vi "Insert Data Point.vi"(4 "Error In":errorcluster, 6 "Instance Name":T1, 7 "Data":T2) -> (0 "Error Out":errorcluster)   [LabVIEW 2015, in "Temperature Controller Data Buffer.lvlib"]
uses:
  Temperature Controller Data Buffer.lvlib
  _libraries/Startup Processes/_typedefs/Subpanel Names.ctl
  _libraries/Startup Processes/Startup Processes.lvlib
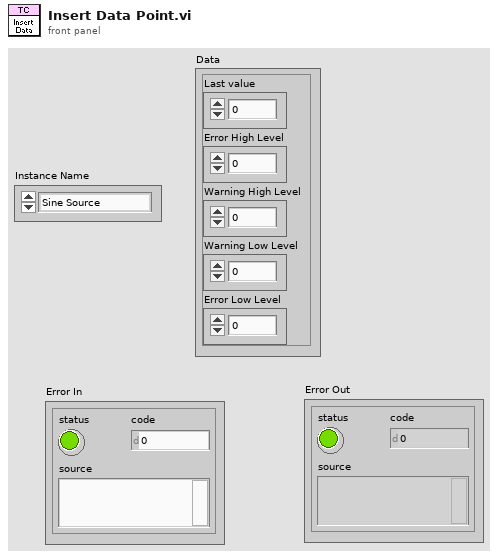
[diagram p1: front panel]
types:
  T1 = typedef "Startup Processes.lvlib/Subpanel Names.ctl" = enum16{"Sine Source", "Ramp Source", "Hen House TC", "Dog House TC", "Out House TC"}
  T2 = cluster{"Last value":dbl, "Error High Level":dbl, "Warning High Level":dbl, "Warning Low Level":dbl, "Error Low Level":dbl}
  T3 = typedef "Temperature Controller Data Buffer.lvlib/buffer data typedef.ctl" = cluster{"TC Data":cluster{"Last value":dbl, "Error High Level":dbl, "Warning High Level":dbl, "Warning Low Level":dbl, "Error Low Level":dbl}[], "Counter":i32}
  T4 = cluster{"Last value":dbl, "Error High Level":dbl, "Warning High Level":dbl, "Warning Low Level":dbl, "Error Low Level":dbl}[]
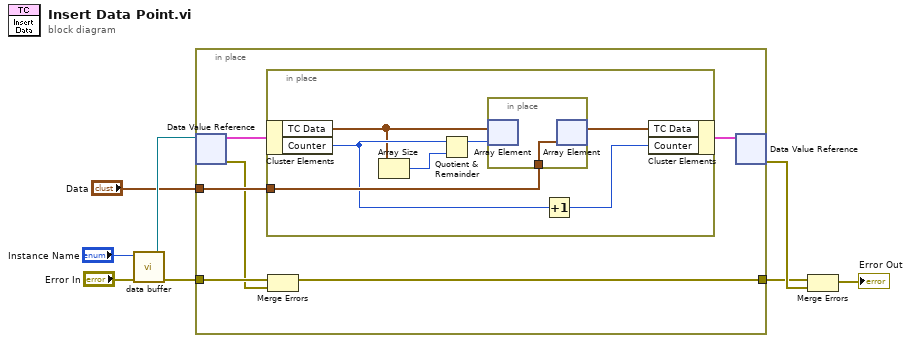
[diagram p0: block diagram]
diagram:
  n1 = call "data buffer.vi"("Error In"="Error In", "Instance Name"="Instance Name") -> ("Error Out"=w3:errorcluster, "DVR"=w7:refnum<data-value>)  [unwired: 4 in]
  n2 = in-place {
    in-place-border: "Data" -> [w12]
    in-place-border: w3 -> [w11]
    in-place-border: [w9] -> w2
    n3 = in-place-dvr #1(w7) -> (w14:T3, w10:errorcluster)
    n4 = in-place {
      in-place-border: w12 -> [w21]
      n5 = in-place-cluster #2(w14) -> ("TC Data"=w15:T4, "Counter"=w18:i32)
      n6 = Array Size(array=w15) -> (size(s)=w16:i32)
      n7 = Quotient & Remainder(x=w18, y=w16) -> (x-y*floor(x/y)=w19:i32)  [unwired: 1 out]
      n8 = in-place {
        in-place-border: w21 -> [w22]
        n9 = in-place-array #3(w15, w19) -> ()  [unwired: 1 out]
        n10 = in-place-array #3(w22) -> (w20:T4)  [unwired: 1 out]
      }
      n11 = Increment(x=w18) -> (x+1=w17:i32)
      n12 = in-place-cluster #2("TC Data"=w20, "Counter"=w17) -> (w13:T3)
    }
    n13 = Merge Errors(w11, w10) -> (w9:errorcluster)
    n14 = in-place-dvr #1(w13) -> (w4:errorcluster)  [unwired: 1 out]
  }
  n15 = Merge Errors(w2, w4) -> (→"Error Out":errorcluster)
